vi "Save_Max_and_Min_Values.vi"() -> (5 "Plug in titles":string[](array[string]), 7 "Plug in values":string[](array[string]))   [LabVIEW 2012]
uses:
  Globals/Meas_global.vi
panel:
  in  "No of Points to average over":i32=2 min=1 step=1
  out "Minimums":dbl[](array[numeric]) format="%.2f"
  out "Maximums":dbl[](array[numeric]) format="%.2f"
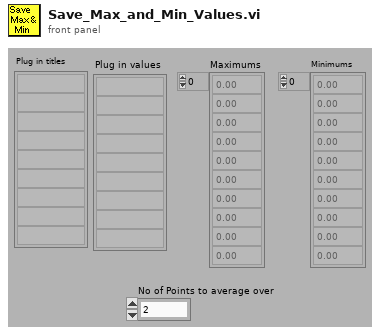
[diagram p1: front panel]
types:
  T1 = typedef "Analysis_info_cluster.ctl" = cluster{"Colour":u32, "Inst type":T2, "Inst name":string, "Symbol":string, "Code name":string, "Extra Info":string, "Inst Array":T3, "Extra Titles":string[], "Extra Values":string[], "U":dbl, "u^2":dbl, "u^3":dbl, "u^4":dbl, "Skew_u":dbl, "Kurt_u":dbl, "Sd Error in Mean":dbl, "% u'/U":dbl, "X":dbl, "Y":dbl, "Z":dbl, "Timescale integral to 25%":dbl, "Sd Error in Variance":dbl, "Calib File":path, "Calib Constants":dbl[], "Output Position":bool, "Full Stats":bool, "Av Sampling Rate":dbl, "Av No of Samples":dbl, "Total Meas Time (s)":dbl, "ADAM Ch Name":string}
  T2 = typedef "Inst_type.ctl" = enum16{"Propeller anemometer", "Raw voltage", "Pressure Transducer", "Pitot-static tube", "Preston tube", "Hot wire", "Cross wire 1", "Cross wire 2", "Generic Linear", "Generic Polynomial", "Generic BackPoly", "Fast FID", "Thermocouple", "Cold wire", "Pulsed Wire", "LDA Vel", "LDA Tran time", "LDA Arr time"}
  T3 = typedef "Instrument_Array.ctl" = enum16{"PWA", "LDA", "Analogue"}
  T4 = typedef "Time_Trace_Cluster.ctl" = cluster{"Weighting":dbl[], "Time (s)":dbl[], "Voltage":dbl[], "Eng Values":dbl[]}
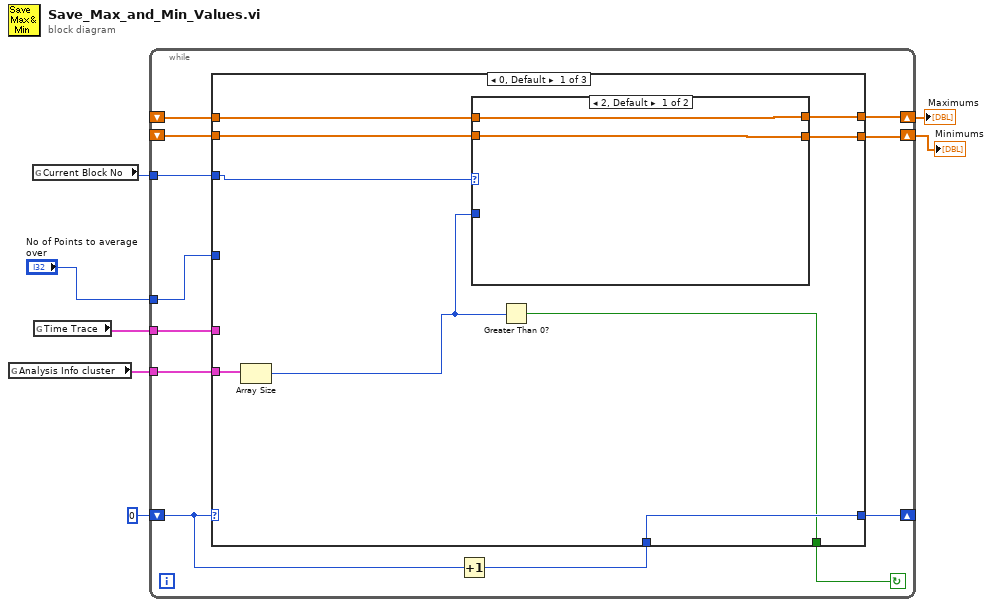
[diagram p0: block diagram]
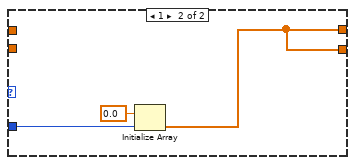
[diagram p2: hidden frame]
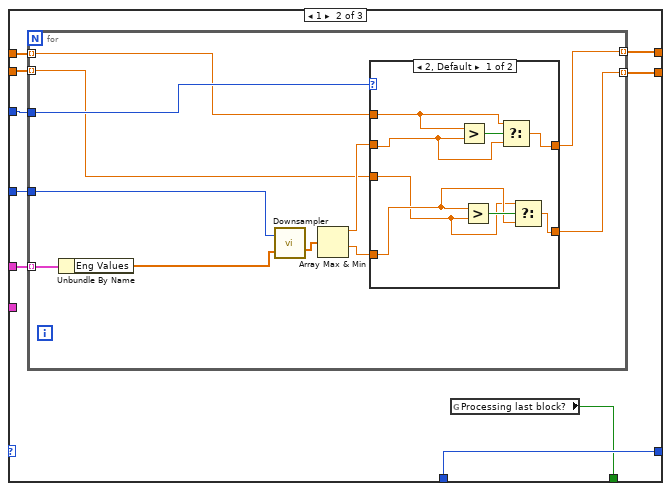
[diagram p3: hidden frame]
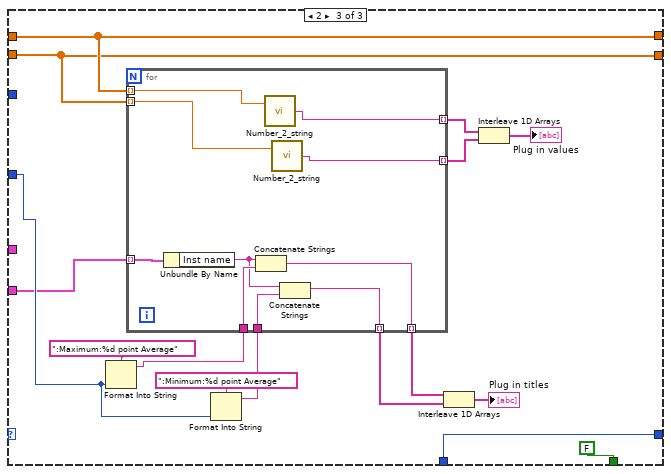
[diagram p5: hidden frame]
diagram:
  n1 = global read "Meas_global.vi" "Analysis Info cluster"() -> (w2:T1[])
  n2 = global read "Meas_global.vi" "Current Block No"() -> (w7:i32)
  n3 = global read "Meas_global.vi" "Time Trace"() -> (w1:T4[])
  n4 = while {
    shift-left: _ -> [w13]
    shift-right: [w14] -> w5
    shift-left: _ -> [w11]
    shift-right: [w12] -> w4
    shift-left: 0 -> [w18]
    shift-right: [w16] -> _
    tunnel: w7 -> [w19]
    tunnel: "No of Points to average over" -> [w10]
    tunnel: w2 -> [w9]
    tunnel: w1 -> [w8]
    stop <- w15 continue-if-true
    n5 = Increment(x=w18) -> (x+1=w17:i32)
    n6 = case shown="0, Default" w18 {
      tunnel: w19 -> [w26 w42 _]
      tunnel: w17 -> [w28 w41 w78]
      tunnel: [w28 w41 w78] -> w16
      tunnel: [w27 w36 FALSE] -> w15
      tunnel: [w25 w38 w71] -> w14
      tunnel: w13 -> [w24 w40 w71]
      tunnel: [w23 w37 w70] -> w12
      tunnel: w11 -> [w22 w39 w70]
      tunnel: w10 -> [_ w35 w67]
      tunnel: w9 -> [w21 _ w64]
      tunnel: w8 -> [_ w34 _]
      frame 0, Default {
        n7 = Array Size(array=w21) -> (size(s)=w20:i32)
        n8 = case shown="2, Default" w26 {
          tunnel: [w30 w31] -> w25
          tunnel: w24 -> [w30 _]
          tunnel: [w29 w31] -> w23
          tunnel: w22 -> [w29 _]
          tunnel: w20 -> [_ w33]
          frame 2, Default {
          }
          frame 1 {
            n9 = Initialize Array(0.0 ("Element Data"), w33) -> (w31:dbl[])
          }
        }
        n10 = Greater Than 0?(x=w20) -> (x > 0?=w27:bool)
      }
      frame 1 {
        n11 = for {
          tunnel: w42 -> [w51]
          tunnel: w40 -> [w50] mode=indexing
          tunnel: w39 -> [w49] mode=indexing
          tunnel: [w48] -> w38 mode=indexing
          tunnel: [w47] -> w37 mode=indexing
          tunnel: w35 -> [w45]
          tunnel: w34 -> [w44] mode=indexing
          n12 = Unbundle By Name(w44) -> ("Eng Values"=w43:dbl[])
          n13 = call "Downsampler.vi"("Input Array"=w43, "Averaging samples"=w45) -> ("Downsampled Array"=w46:dbl[])  [unwired: 1 out]
          n14 = Array Max & Min(array=w46) -> (max value=w53:dbl, min value=w52:dbl)  [unwired: 2 out]
          n15 = case shown="2, Default" w51 {
            tunnel: [w59 w63] -> w48
            tunnel: w53 -> [w60 w63]
            tunnel: [w56 w62] -> w47
            tunnel: w52 -> [w57 w62]
            tunnel: w50 -> [w55 _]
            tunnel: w49 -> [w54 _]
            frame 2, Default {
              n16 = Greater?(x=w55, y=w60) -> (0:w61:bool)
              n17 = Greater?(x=w57, y=w54) -> (0:w58:bool)
              n18 = Select(t=w55, s=w61, f=w60) -> (s? t:f=w59:dbl)
              n19 = Select(t=w54, s=w58, f=w57) -> (s? t:f=w56:dbl)
            }
            frame 1 {
            }
          }
        }
        n20 = global read "Meas_global.vi" "Processing last block?"() -> (w36:bool)
      }
      frame 2 {
        n21 = Format Into String(format string=":Maximum:%d point Average", w67) -> (resulting string=w65:string)  [unwired: 2 in, 1 out]
        n22 = Format Into String(format string=":Minimum:%d point Average", w67) -> (resulting string=w66:string)  [unwired: 2 in, 1 out]
        n23 = for {
          tunnel: w64 -> [w89] mode=indexing
          tunnel: w65 -> [w88]
          tunnel: w66 -> [w86]
          tunnel: [w85] -> w77 mode=indexing
          tunnel: [w84] -> w76 mode=indexing
          tunnel: w71 -> [w83] mode=indexing
          tunnel: w70 -> [w82] mode=indexing
          tunnel: [w80] -> w74 mode=indexing
          tunnel: [w81] -> w73 mode=indexing
          n24 = Unbundle By Name(w89) -> ("Inst name"=w87:string)
          n25 = Concatenate Strings(w87, w88) -> (w85:string)
          n26 = call "Number_2_string.vi"("number"=w83) -> ("String"=w80:string)  [unwired: 1 in]
          n27 = call "Number_2_string.vi"("number"=w82) -> ("String"=w81:string)  [unwired: 1 in]
          n28 = Concatenate Strings(w87, w86) -> (w84:string)
        }
        n29 = Interleave 1D Arrays(w77, w76) -> (→"Plug in titles":string[])
        n30 = Interleave 1D Arrays(w74, w73) -> (→"Plug in values":string[])
      }
    }
  }
  "Maximums" <- w5
  "Minimums" <- w4
